vi "PH_Tektronix_7000.set modified data.vi"(0 "i ref in":refnum<vi>, 2 "i attribute":T1={"VISA Resource Name"="GPIB0::1::INSTR", "IDN"={"Instrument Driver"="", "Instrument Firmware"="", "Model"="", "Serial Number"=""}, "Selftest"={"Result"=0, "Message"="N/A"}, "Trigger Configuration"={"Source"=0, "Level [V]"=0.0, "Slope"=0, "Coupling"=0, "Trigger Mode"=0}, "Acquisition Configuration"={"Record Length"=10000, "Timebase [s/div]"=4.0, "Position [%]"=0.0, "Acquisition Type"=0, "Average Waveforms"=10, "Envelope Waveforms"=10, "WfmDB Samples"=16000, "Continuous?"=FALSE, "Delay [s]"=0.0, "Run?"=FALSE}, "GUI Refs"={"Graph"=refnum, "State"=refnum, "Delete"=refnum, "VISA Resource"=refnum, "Allow Configure"=refnum, "Fetch Data"=refnum, "Fetch before sending Data to PSDB"=refnum, "Name Channel 1"=refnum, "Name Channel 2"=refnum, "Name Channel 3"=refnum, "Name Channel 4"=refnum, "Prdc Intervall [ms]"=refnum, "Data taken"=refnum, "Model"=refnum, "Serial Number"=refnum, "Firmware"=refnum, "Driver"=refnum, "Acquisition"=refnum, "Trigger"=refnum, "Cursor: D Time [s]"=refnum, "Cursor: D Signal [V]"=refnum, "Channel 1"=refnum, "Channel 2"=refnum, "Channel 3"=refnum, "Channel 4"=refnum}, "State"=0, "Error Message"="", "Allow Prdc Loop?"=FALSE, "Channel 1"={"Enable Channel"=FALSE, "Bandwidth"=0, "Input Impedance"=0, "Vertical Coupling"=0, "Probe Attenuation"=1.0, "Range [V/div]"=1.0, "Position [div]"=10.0, "Bandwidth raw"=""}, "Channel 2"={"Enable Channel"=FALSE, "Bandwidth"=0, "Input Impedance"=0, "Vertical Coupling"=0, "Probe Attenuation"=1.0, "Range [V/div]"=1.0, "Position [div]"=10.0, "Bandwidth raw"=""}, "Channel 3"={"Enable Channel"=FALSE, "Bandwidth"=0, "Input Impedance"=0, "Vertical Coupling"=0, "Probe Attenuation"=1.0, "Range [V/div]"=1.0, "Position [div]"=10.0, "Bandwidth raw"=""}, "Channel 4"={"Enable Channel"=FALSE, "Bandwidth"=0, "Input Impedance"=0, "Vertical Coupling"=0, "Probe Attenuation"=1.0, "Range [V/div]"=1.0, "Position [div]"=10.0, "Bandwidth raw"=""}, "Data CH 1"={"t0"=timestamp(3.694502999999883e-07 s since 1904-01-01), "dt"=5e-07, "Y"=array[10000 elements]}, "Data CH 2"={"t0"=timestamp(3.694502999999883e-07 s since 1904-01-01), "dt"=5e-07, "Y"=array[10000 elements]}, "Data CH 3"={"t0"=timestamp(3.694502999999883e-07 s since 1904-01-01), "dt"=5e-07, "Y"=array[10000 elements]}, "Data CH 4"={"t0"=timestamp(3.694502999999883e-07 s since 1904-01-01), "dt"=5e-07, "Y"=array[10000 elements]}, "Allow config?"=FALSE, "Name Channel 1"="", "Name Channel 2"="", "Name Channel 3"="", "Name Channel 4"="", "Fetch Data before sending to PSDB?"=FALSE, "Constructor passed?"=FALSE, "Data taken at"=timestamp(0 s since 1904-01-01), "Plot Colors"=[], "Default VISA Resource"=""} {"Channel 4"."Vertical Coupling" items=["AC", "DC", "Ground"]; "Channel 4"."Input Impedance" items=["1M", "50"]; "Channel 4"."Bandwidth" items=["FULL", "500 MHz", "250 MHz", "150 MHz", "20 MHz"]; "Channel 3"."Vertical Coupling" items=["AC", "DC", "Ground"]; "Channel 3"."Input Impedance" items=["1M", "50"]; "Channel 3"."Bandwidth" items=["FULL", "500 MHz", "250 MHz", "150 MHz", "20 MHz"]; "Channel 2"."Vertical Coupling" items=["AC", "DC", "Ground"]; "Channel 2"."Input Impedance" items=["1M", "50"]; "Channel 2"."Bandwidth" items=["FULL", "500 MHz", "250 MHz", "150 MHz", "20 MHz"]; "Channel 1"."Vertical Coupling" items=["AC", "DC", "Ground"]; "Channel 1"."Input Impedance" items=["1M", "50"]; "Channel 1"."Bandwidth" items=["FULL", "500 MHz", "250 MHz", "150 MHz", "20 MHz"]; "State" items=["no info", "off/false/out", "on/true/in", "Failure", "Alarm", "Status 1", "Status 2", "Status 3"]; "Acquisition Configuration"."Delay [s]" format="%#_12p"; "Acquisition Configuration"."Acquisition Type" items=["Sample", "Peak Detect", "Hi Res", "Average", "Envelope", "WfmDB"]; "Acquisition Configuration"."Timebase [s/div]" format="%#_12g"; "Trigger Configuration"."Trigger Mode" items=["Normal", "Auto"]; "Trigger Configuration"."Coupling" items=["DC", "AC", "Hf Reject", "Lf Reject", "Noise Rej", "Atrigger"]; "Trigger Configuration"."Slope" items=["Rise", "Fall", "Either"]; "Trigger Configuration"."Source" items=["Channel1"=0, "Channel2"=1, "Channel3"=2, "Channel4"=3, "Aux"=12, "Line"=13]; "Selftest"."Result" format="%.0x"}, 5 "error in (no error)":errorcluster) -> (14 "i ref out":refnum<vi>, 19 "error out":errorcluster)   [LabVIEW 2014, in "PH_Tektronix_7000.lvlib"]
doc: "Writes the data into the attribute of an object. Then, the attribute dara are unlocked using the \"release\" method. Prior to calling THIS method, the attribute data must have been locked using the methods \"lock\" or \"get data to modify\".\n\n\nLicense Agreement for this software:\n\nCopyright (C)\nGesellschaft für Schwerionenforschung, GSI\nPlanckstr. 1\n64291 Darmstadt\nGermany\n\nContact: D.Beck@gsi.de \n\nThis program is free software; you can redistribute it and/or modify it under the terms of the GNU General Public License as published by the Free Software Foundation; either version 2 of the license, or (at your option) any later version.\n\nThis program is distributed in the hope that it will be useful, but WITHOUT ANY WARRANTY; without even the implied warranty of MERCHANTABILITY or FITNESS FOR A PARTICULAR PURPOSE. See the GNU General License for more details (http://www.gnu.org).\n\nGesellschaft für Schwerionenforschung, GSI\nPlanckstr. 1, 64291 Darmstadt, Germany\nFor all questions and ideas contact: M.Richter@gsi.de, H.Brand@gsi.de or D.Beck@gsi.de.\nLast update: 17-JUN-2004"
uses:
  PH_Tektronix_7000.lvlib
  PH_Tektronix_7000.i attribute.ctl
  PH_Tektronix_7000.Trigger Config.ctl
  PH_Tektronix_7000.Acquisition Config.ctl
  PH_Tektronix_7000.GUI Refs.ctl
  PH_StatusHandler/PH_StatusHandler.Status.ctl
  PH_Tektronix_7000.Channel Config.ctl
  CSCore/CSObj/CSObj.lvlib
  PH_StatusHandler/PH_StatusHandler.lvlib
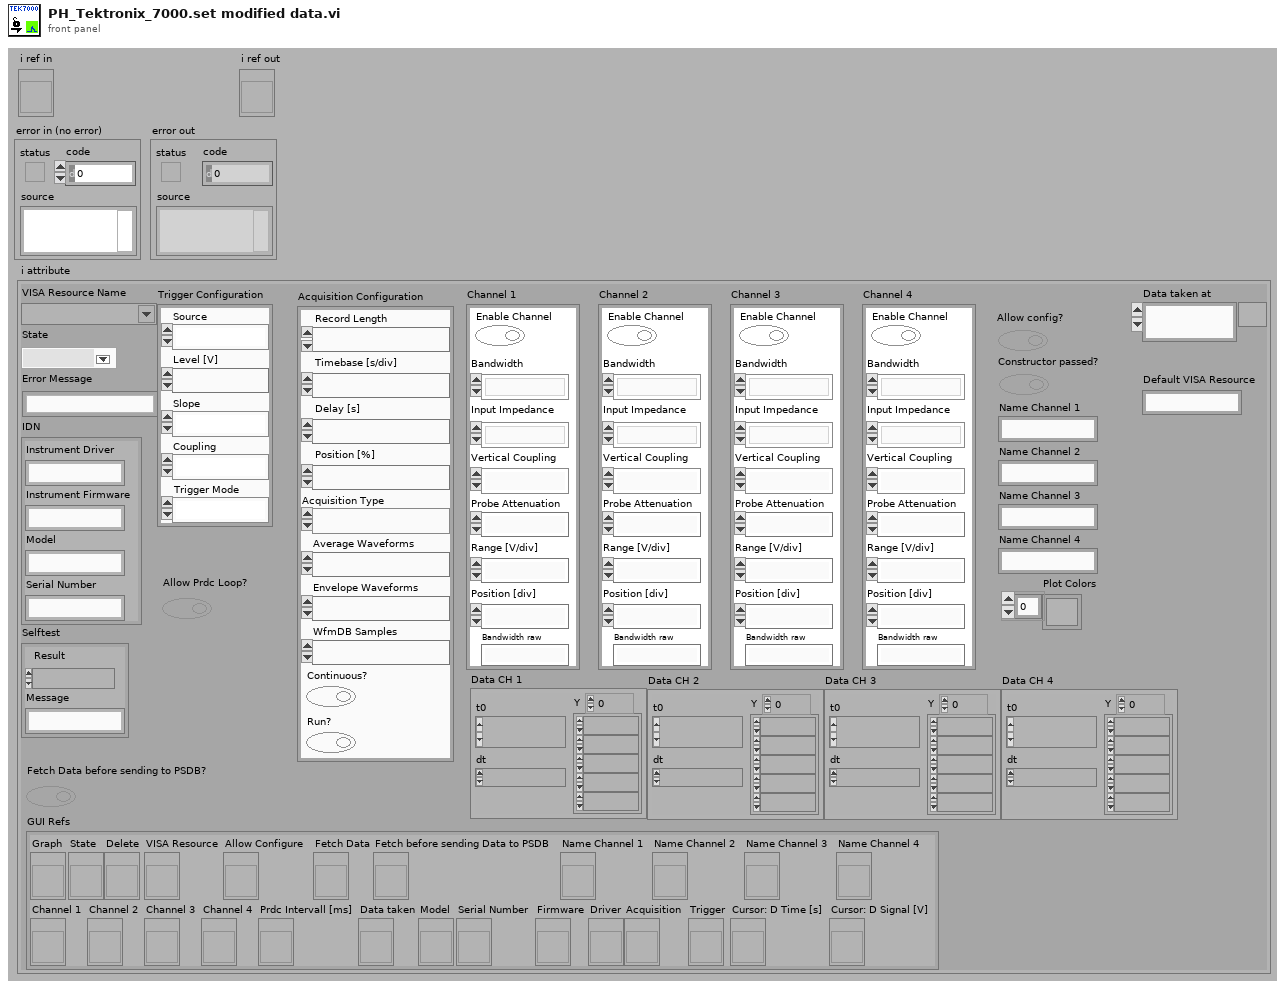
[diagram p1: front panel]
types:
  T1 = typedef "PH_Tektronix_7000.lvlib/PH_Tektronix_7000.i attribute.ctl" = cluster{"VISA Resource Name":refnum<visa-resource-name>, "IDN":cluster{"Instrument Driver":string, "Instrument Firmware":string, "Model":string, "Serial Number":string}, "Selftest":cluster{"Result":i32, "Message":string}, "Trigger Configuration":T2, "Acquisition Configuration":T3, "GUI Refs":T4, "State":T5, "Error Message":string, "Allow Prdc Loop?":bool, "Channel 1":T6, "Channel 2":T6, "Channel 3":T6, "Channel 4":T6, "Data CH 1":waveform(dbl), "Data CH 2":waveform(dbl), "Data CH 3":waveform(dbl), "Data CH 4":waveform(dbl), "Allow config?":bool, "Name Channel 1":string, "Name Channel 2":string, "Name Channel 3":string, "Name Channel 4":string, "Fetch Data before sending to PSDB?":bool, "Constructor passed?":bool, "Data taken at":timestamp, "Plot Colors":u32[], "Default VISA Resource":string}
  T2 = typedef "PH_Tektronix_7000.lvlib/PH_Tektronix_7000.Trigger Config.ctl" = cluster{"Source":u16, "Level [V]":dbl, "Slope":u16, "Coupling":u16, "Trigger Mode":u16}
  T3 = typedef "PH_Tektronix_7000.lvlib/PH_Tektronix_7000.Acquisition Config.ctl" = cluster{"Record Length":u32, "Timebase [s/div]":dbl, "Position [%]":dbl, "Acquisition Type":u16, "Average Waveforms":i32, "Envelope Waveforms":i32, "WfmDB Samples":i32, "Continuous?":bool, "Delay [s]":dbl, "Run?":bool}
  T4 = typedef "PH_Tektronix_7000.lvlib/PH_Tektronix_7000.GUI Refs.ctl" = cluster{"Graph":refnum<vi>, "State":refnum<vi>, "Delete":refnum<vi>, "VISA Resource":refnum<vi>, "Allow Configure":refnum<vi>, "Fetch Data":refnum<vi>, "Fetch before sending Data to PSDB":refnum<vi>, "Name Channel 1":refnum<vi>, "Name Channel 2":refnum<vi>, "Name Channel 3":refnum<vi>, "Name Channel 4":refnum<vi>, "Prdc Intervall [ms]":refnum<vi>, "Data taken":refnum<vi>, "Model":refnum<vi>, "Serial Number":refnum<vi>, "Firmware":refnum<vi>, "Driver":refnum<vi>, "Acquisition":refnum<vi>, "Trigger":refnum<vi>, "Cursor: D Time [s]":refnum<vi>, "Cursor: D Signal [V]":refnum<vi>, "Channel 1":refnum<vi>, "Channel 2":refnum<vi>, "Channel 3":refnum<vi>, "Channel 4":refnum<vi>}
  T5 = typedef "PH_StatusHandler.lvlib/PH_StatusHandler.Status.ctl" = i16
  T6 = typedef "PH_Tektronix_7000.lvlib/PH_Tektronix_7000.Channel Config.ctl" = cluster{"Enable Channel":bool, "Bandwidth":u16, "Input Impedance":u16, "Vertical Coupling":u16, "Probe Attenuation":dbl, "Range [V/div]":dbl, "Position [div]":dbl, "Bandwidth raw":string}
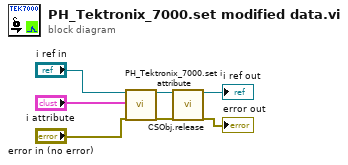
[diagram p0: block diagram]
diagram:
  n1 = call "PH_Tektronix_7000.set i attribute.vi"("i ref in"="i ref in", "i attribute"="i attribute", "error in (no error)"="error in (no error)") -> ("i ref out"=w4:refnum<vi>, "error out"=w3:errorcluster)  [unwired: 15 in]
  n2 = call "CSObj.release.vi"("i ref in"=w4, "error in (no error)"=w3) -> ("i ref out"=→"i ref out":refnum<vi>, "error out"=→"error out":errorcluster)  [unwired: 16 in]
